vi "Acquisition-START case.vi"(10 "Acquired z-plane index":i32, 11 "Message Queues":T1) -> (0 "error out":errorcluster, 2 "Index of z-plane to acquire next":i32)   [LabVIEW 2020]
uses:
  User Interface/Queue/Message Queue/Typedefs/All Message Queues.ctl
  User Interface/Queue/Message Queue/Typedefs/Message Cluster.ctl
  Typedefs/Logging queue element.ctl
  Typedefs/Imaging Protocols enum.ctl
  Typedefs/Frame Size.ctl
  Typedefs/Acquired points count.ctl
  Typedefs/Read Write Enum.ctl
  Global Variables/General Globals.vi
panel:
  in  "error in":errorcluster
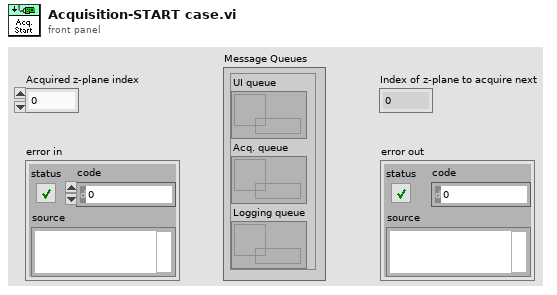
[diagram p1: front panel]
types:
  T1 = typedef "All Message Queues.ctl" = cluster{"UI queue":refnum<queue>, "Acq. queue":refnum<queue>, "Logging queue":refnum<queue>}
  T2 = enum8{"Enabled", "Disabled", "Disabled and Grayed Out"}
  T3 = typedef "Read Write Enum.ctl" = enum16{"Read", "Write"}
  T4 = typedef "AOL_Globals.ctl" = cluster{"Imaging Protocol":T5, "Number of POI":u16, "Number of Miniscans":u16, "Number of Trials":u16, "Number of Cycles ":u64, "# Averaged Frames":u16, "Laser power (%)":u8, "Pockels (V)":dbl, "Acquisition Length (sec)":dbl, "Fill time (us)":dbl, "POI Dwell time (us)":dbl, "Miniscan Dwell time per pixel (us)":dbl, "PMT 1":dbl, "PMT 2":dbl, "Back Apperture (mA)":dbl, "Frame Size":T6, "Center Frequency":dbl, "Field of View (norm)":dbl, "DwellTime (us)":dbl, "Wavelength (nm)":dbl, "Zoom":dbl, "AOL Z":dbl, "AOL Mode":T7, "GridXY":dbl, "GridZ":dbl, "TriggerPeriod (sec)":dbl, "Number of Pixels in Miniscan":u16, "Experiment folder path":path, "X centre":dbl, "Y centre":dbl, "Angle (degrees)":dbl, "Plane Mode":T8, "Threshold":u16[], "Regenerate Chirps":bool, "Rectangle ROI length (pixels)":u16, "Rectangle ROI height (pixels)":u16, "AOD fill":u16, "StartupDelay":i32, "Samples Wait after Trigger":u16, "Slip Cycle":u32, "Add Cycle":bool, "Functional Mode":T9, "Z Start":dbl, "Z Stop":dbl, "# Planes":i32, "Total Pixels":i32, "Variable Miniscan Pixels":u16[], "Use Variable Length":bool, "Use Variable Resolution":bool, "Laser power (%) at Z Start":u8, "Laser power (%) at Z Stop":u8, "Ref Z Step":i8, "Ref Dwell Time (us)":dbl, "Field of View (um)":dbl}
  T5 = typedef "Imaging Protocols enum.ctl" = enum16{"AOL Z-Stack", "Motor Z Stack", "Functional Acquisition", "Single Plane Acquisition", "Volume Acquisition", "Live Imaging", "Live Plane Imaging", "Live Volume Imaging"}
  T6 = typedef "Frame Size.ctl" = u16
  T7 = typedef "AOL modes.ctl" = enum16{"Raster", "Structural", "Pointing", "Mini Scan", "Alignment"}
  T8 = typedef "Plane Mode.ctl" = u16
  T9 = typedef "Functional Mode.ctl" = enum16{"Point", "Line", "Patch", "Plane", "Volume"}
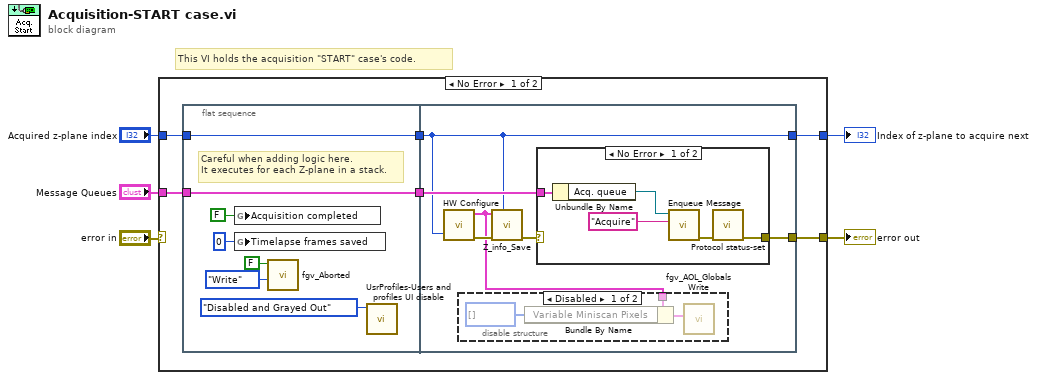
[diagram p0: block diagram]
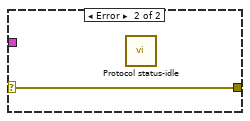
[diagram p3: hidden frame]
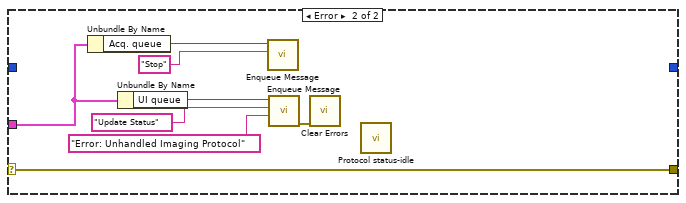
[diagram p4: hidden frame]
diagram:
  # "This VI holds the acquisition \"START\" case's code."
  n1 = case shown="No Error" "error in" {
    selector: "error in" -> [_ w35]
    tunnel: [w11 w35] -> w3
    tunnel: [w8 _] -> w4
    tunnel: "Message Queues" -> [w9 w34]
    tunnel: "Acquired z-plane index" -> [w10 _]
    frame No Error {
      n2 = flat-sequence {
        tunnel: w9 -> [w17]
        tunnel: w10 -> [w18]
        tunnel: [w18] -> w7
        tunnel: [w17] -> w6
        tunnel: [w24] -> w11
        tunnel: [w21] -> w8
        tunnel: w7 -> [w21]
        tunnel: w6 -> [w22]
        frame #0 {
          # "Careful when adding logic here.\nIt executes for each Z-plane in a stack."
          n3 = global write "General Globals.vi" "Acquisition completed"(FALSE ("Acquisition completed")) -> ()
          n4 = global write "General Globals.vi" "Timelapse frames saved"(u32 0 ("Timelapse frames saved")) -> ()
          n5 = call "fgv_Aborted.vi"("Function"=Read_Write_Enum."Write", "Funct Acq Aborted"=FALSE ("Aborted acquisition")) -> ()  [unwired: 8 in, 2 out]
          n6 = call "UsrProfiles-Users and profiles UI disable.vi"("Users & Profiles available?"=T2."Disabled and Grayed Out") -> ()  [unwired: 10 in, 1 out]
        }
        frame #1 {
          n7 = call "HW Configure.vi"("Acquired z-plane index"=w21) -> ("Error Out"=w23:errorcluster, "AOL_Globals"=w19:T4)  [unwired: 9 in]
          n8 = disable-structure shown="Disabled" {
            disable-tunnel: w19 -> [w27 _]
            frame Disabled {
              n9 = Bundle By Name(cluster=w27, "Variable Miniscan Pixels"=u16[] []) -> (w26:T4)
              n10 = call "fgv_AOL_Globals Write.vi"("AOL_Globals"=w26) -> ()  [unwired: 10 in, 1 out]
            }
            frame Enabled {
            }
          }
          n11 = call "Z_info_Save.vi"("Zplane in"=w21, "error in (no error)"=w23, "AOL_Globals"=w19) -> ("error out"=w20:errorcluster)  [unwired: 8 in]
          n12 = case shown="No Error" w20 {
            selector: w20 -> [_ w33]
            tunnel: [w28 w33] -> w24
            tunnel: w22 -> [w30 _]
            frame No Error {
              n13 = Unbundle By Name(w30) -> ("Acq. queue"=w32:refnum<queue>)
              n14 = call "Enqueue Message.vi"("Message"="Acquire", "Queue"=w32) -> ("error out"=w29:errorcluster)  [unwired: 8 in, 1 out]
              n15 = call "Protocol status-set.vi"("error in"=w29) -> ("error out"=w28:errorcluster)  [unwired: 10 in]
            }
            frame Error {
              n16 = call "Protocol status-idle.vi"() -> ()  [unwired: 12 in]
            }
          }
        }
      }
    }
    frame Error {
      n17 = Unbundle By Name(w34) -> ("Acq. queue"=w39:refnum<queue>)
      n18 = Unbundle By Name(w34) -> ("UI queue"=w40:refnum<queue>)
      n19 = call "Enqueue Message.vi"("Message"="Stop", "Queue"=w39) -> ()  [unwired: 8 in, 2 out]
      n20 = call "Enqueue Message.vi"("Message Data"="Error: Unhandled Imaging Protocol" ("Message"), "Message"="Update Status", "Queue"=w40) -> ("error out"=w36:errorcluster)  [unwired: 7 in, 1 out]
      n21 = call <vilib>:"Clear Errors.vi"("error in (no error)"=w36) -> ()  [unwired: 5 in, 2 out]
      n22 = call "Protocol status-idle.vi"() -> ()  [unwired: 12 in]
    }
  }
  "Index of z-plane to acquire next" <- w4
  "error out" <- w3
